vi "Sensor.vi"(0 "VISA resource name":refnum<visa-resource-name>="GPIB0::12::INSTR", 5 "Channel (1)":dbl, 11 "error in (no error)":errorcluster) -> (4 "VISA resource name out":refnum<visa-resource-name>="COM1", 6 "Resistance Reading":dbl min=0.0 max=63200000.0 step=1e-05 format="%^.5e", 8 "Kelvin Reading":dbl min=0.0 max=1000.0 step=1e-05 format="%^.5e", 10 "Power Reading":dbl min=0.0 max=0.01 step=1e-05 format="%^.5e", 15 "error out":errorcluster={"status"=TRUE, "code"=-1073807339, "source"="VISA Read in Lake Shore Cryotronics 370.lvlib:Sensor.vi"})   [LabVIEW 2014, in "Lake Shore Cryotronics 370.lvlib"]
doc: "This VI querys the instrument for an channels's sensor reading in Resistance, Kelvin, and Power."
uses:
  <instrlib>/Lake Shore Cryotronics 370/Lake Shore Cryotronics 370.lvlib
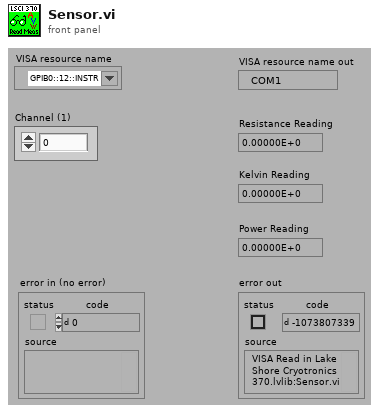
[diagram p1: front panel]
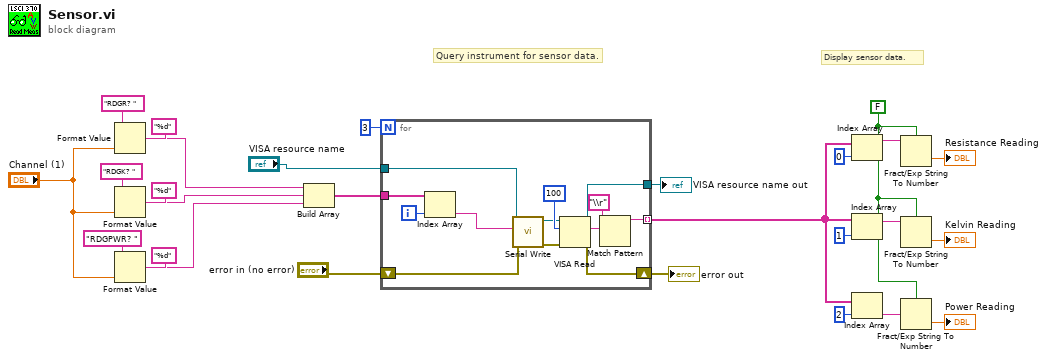
[diagram p0: block diagram]
diagram:
  w15 = FALSE ("use system decimal point (T)")
  # "Display sensor data."
  # "Query instrument for sensor data."
  n1 = Format Value(string ("")="RDGR? ", format string="%d", value (0)="Channel (1)") -> (output string=w8:string)
  n2 = Format Value(string ("")="RDGK? ", format string="%d", value (0)="Channel (1)") -> (output string=w7:string)
  n3 = Format Value(string ("")="RDGPWR? ", format string="%d", value (0)="Channel (1)") -> (output string=w6:string)
  n4 = Build Array(w8, w7, w6) -> (w21:string[])
  n5 = for {
    N: 3 -> [_]
    tunnel: w21 -> [w37]
    shift-right: [w34] -> w18
    shift-left: "error in (no error)" -> [w35]
    tunnel: [w33] -> w17
    tunnel: "VISA resource name" -> [w32]
    tunnel: [w30] -> w16 mode=indexing
    i -> [w36]
    n6 = Index Array(array=w37, index=w36) -> (element=w28:string)
    n7 = call <instrlib>:"Serial Write.vi"("error in (no error)"=w35, "Write Buffer (\"\")"=w28, "VISA resource name"=w32) -> ("error out"=w40:errorcluster, "VISA resource name out"=w29:refnum<visa-resource-name>)  [unwired: 6 in, 1 out]
    n8 = VISA Read(VISA resource name=w29, byte count=100, error in (no error)=w40) -> (VISA resource name out=w33:refnum<visa-resource-name>, read buffer=w38:string, error out=w34:errorcluster)  [unwired: 1 out]
    n9 = Match Pattern(string=w38, regular expression="\\r") -> (before substring=w30:string)  [unwired: 1 in, 3 out]
  }
  "VISA resource name out" <- w17
  "error out" <- w18
  n10 = Index Array(array=w16, index=0) -> (element=w25:string)
  n11 = Index Array(array=w16, index=1) -> (element=w26:string)
  n12 = Index Array(array=w16, index=2) -> (element=w27:string)
  n13 = Fract/Exp String To Number(use system decimal point (T)=w15, string=w25) -> (number=→"Resistance Reading":dbl)  [unwired: 2 in, 1 out]
  n14 = Fract/Exp String To Number(use system decimal point (T)=w15, string=w26) -> (number=→"Kelvin Reading":dbl)  [unwired: 2 in, 1 out]
  n15 = Fract/Exp String To Number(use system decimal point (T)=w15, string=w27) -> (number=→"Power Reading":dbl)  [unwired: 2 in, 1 out]
